vi "Set Cluster Values from Pathed JSON String.vi"(7 "Path":string[](array[string]), 8 "error in (no error)":errorcluster, 10 "JSON string":string, 11 "Clust Refnum":refnum<vi>) -> (0 "error out":errorcluster)   [LabVIEW 2023]
uses:
  <vilib>/Utility/Data Type/NI_Data Type.lvlib
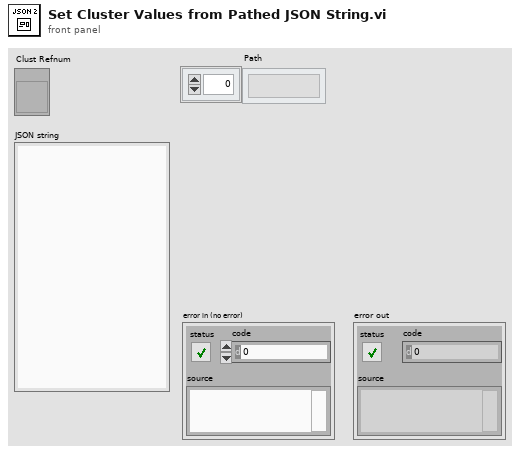
[diagram p1: front panel]
types:
  T1 = typedef "NI_Data Type.lvlib/Data Type.ctl" = enum8{"Invalid Type", "Void", "I8", "I16", "I32", "I64", "U8", "U16", "U32", "U64", "Single Float", "Double Float", "Extended Float", "Single Complex", "Double Complex", "Extended Complex", "Enum U8", "Enum U16", "Enum U32", "Enum U64", "Single Float With Unit", "Double Float With Unit", "Extended Float With Unit", "Single Complex with Unit", "Double Complex with Unit", "Extended Complex with Unit", "Boolean", "String", "Path", "Picture", "Tag", "Array", "Cluster", "Variant", "LV Variant", "Waveform", "Timestamp", "Digital Waveform", "Digital Data", "ExpressData", "Refnum", "External Data", "VI", "Poly VI", "LabVIEW Class Instance", "Fixed Point", "Set Collection", "Map Collection"}
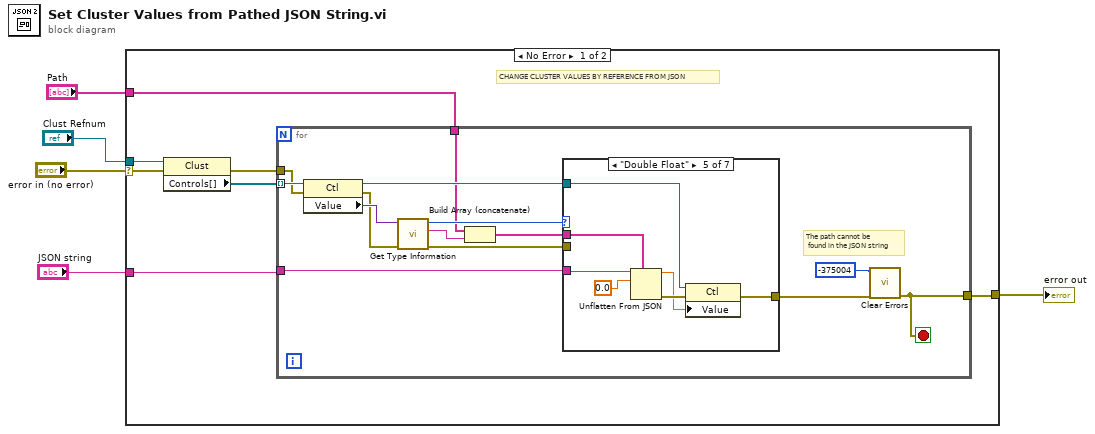
[diagram p0: block diagram]
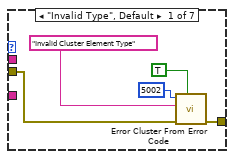
[diagram p2: hidden frame]
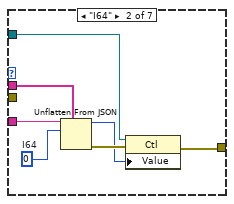
[diagram p3: hidden frame]
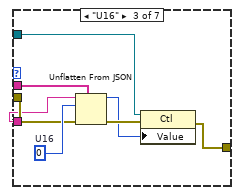
[diagram p4: hidden frame]
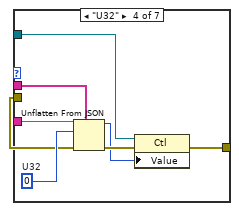
[diagram p5: hidden frame]
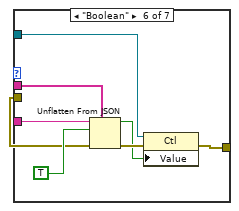
[diagram p6: hidden frame]
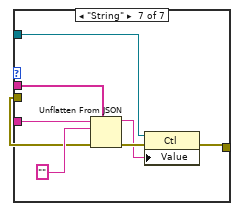
[diagram p7: hidden frame]
diagram:
  n1 = case shown="No Error" "error in (no error)" {
    selector: "error in (no error)" -> [w8 w78]
    tunnel: "Clust Refnum" -> [w10 _]
    tunnel: [w9 w78] -> w5
    tunnel: "JSON string" -> [w7 _]
    tunnel: "Path" -> [w6 _]
    frame No Error {
      # "CHANGE CLUSTER VALUES BY REFERENCE FROM JSON"
      n2 = property class="Clust"(reference=w10, error in=w8) -> (error out=w11:errorcluster, "Controls[]"=w12:refnum<vi>[])  [unwired: 1 out]
      n3 = for {
        tunnel: w7 -> [w26]
        tunnel: w12 -> [w25] mode=indexing
        tunnel: w11 -> [w22]
        tunnel: [w18] -> w9
        tunnel: w6 -> [w14]
        stop <- w18 stop-if-true
        # "The path cannot be\n found in the JSON string"
        n4 = property class="Ctl"(reference=w25, error in=w22) -> (reference out=w19:refnum<vi>, error out=w21:errorcluster, "Value"=w24:variant)
        n5 = call <vilib>:"Get Type Information.vi"("error in (no error)"=w21, "variant"=w24) -> ("error out"=w20:errorcluster, "name"=w13:string, "type"=w23:T1)  [unwired: 5 in, 2 out]
        n6 = Build Array (concatenate)(w14, w13) -> (w15:string[])
        n7 = case shown="\"Double Float\"" w23 {
          tunnel: w26 -> [_ w36 w42 w53 w60 w67 w73]
          tunnel: w15 -> [_ w37 w41 w52 w59 w66 w72]
          tunnel: w20 -> [w28 _ w43 w51 _ w68 w74]
          tunnel: w19 -> [_ w34 w39 w47 w57 w64 w71]
          tunnel: [w31 w32 w40 w48 w55 w62 w70] -> w16
          frame "Invalid Type", Default {
            n8 = call <vilib>:"Error Cluster From Error Code.vi"("show call chain? (False)"=TRUE, "error in (no error)"=w28, "error message (\"\")"="Invalid Cluster Element Type" ("error message (\"\")"), "error code (0)"=5002) -> ("error out"=w31:errorcluster)  [unwired: 5 in]
          }
          frame "I64" {
            w38 = i64 0  # I64
            n9 = Unflatten From JSON(path=w37, JSON string=w36, type and defaults=w38) -> (value=w33:i64, error out=w35:errorcluster)  [unwired: 4 in]
            n10 = property class="Ctl"(reference=w34, error in=w35, "Value"=w33) -> (error out=w32:errorcluster)  [unwired: 1 out]
          }
          frame "U16" {
            w46 = u16 0  # U16
            n11 = Unflatten From JSON(path=w41, JSON string=w42, type and defaults=w46, error in (no error)=w43) -> (value=w44:u16, error out=w45:errorcluster)  [unwired: 3 in]
            n12 = property class="Ctl"(reference=w39, error in=w45, "Value"=w44) -> (error out=w40:errorcluster)  [unwired: 1 out]
          }
          frame "U32" {
            w54 = u32 0  # U32
            n13 = Unflatten From JSON(path=w52, JSON string=w53, type and defaults=w54, error in (no error)=w51) -> (value=w49:u32, error out=w50:errorcluster)  [unwired: 3 in]
            n14 = property class="Ctl"(reference=w47, error in=w50, "Value"=w49) -> (error out=w48:errorcluster)  [unwired: 1 out]
          }
          frame "Double Float" {
            n15 = Unflatten From JSON(path=w59, JSON string=w60, type and defaults=0.0) -> (value=w56:dbl, error out=w58:errorcluster)  [unwired: 4 in]
            n16 = property class="Ctl"(reference=w57, error in=w58, "Value"=w56) -> (error out=w55:errorcluster)  [unwired: 1 out]
          }
          frame "Boolean" {
            n17 = Unflatten From JSON(path=w66, JSON string=w67, type and defaults=TRUE, error in (no error)=w68) -> (value=w63:bool, error out=w65:errorcluster)  [unwired: 3 in]
            n18 = property class="Ctl"(reference=w64, error in=w65, "Value"=w63) -> (error out=w62:errorcluster)  [unwired: 1 out]
          }
          frame "String" {
            n19 = Unflatten From JSON(path=w72, JSON string=w73, type and defaults="", error in (no error)=w74) -> (value=w75:string, error out=w76:errorcluster)  [unwired: 3 in]
            n20 = property class="Ctl"(reference=w71, error in=w76, "Value"=w75) -> (error out=w70:errorcluster)  [unwired: 1 out]
          }
        }
        n21 = call <vilib>:"Clear Errors.vi"("error in (no error)"=w16, "specific error code to clear (0: all)"=-375004) -> ("error out"=w18:errorcluster)  [unwired: 4 in, 1 out]
      }
    }
    frame Error {
    }
  }
  "error out" <- w5
